vi "uTTA_GetLiveMeasureStatus.vi"(4 "CH1&2 Offset Voltage":dbl format="%.3pV", 6 "CH0 Offset Voltage":dbl format="%.3pV", 7 "uTTA_CalData":T1(array[cluster]), 8 "error in":errorcluster, 9 "CalibrationMode":bool, 10 "Timeout(ms)":i32=1000, 11 "VISA Refnum in":refnum<visa-resource-name>) -> (0 "error out":errorcluster, 1 "Measurement Completed":bool, 2 "Received":string, 3 "VISA Refnum out":refnum<visa-resource-name>, 5 "Measurement Data":T3)   [LabVIEW 2021]
uses:
  uTTA_Device_Driver/uTTA_Controls/CTL_uTTA_MeasurementStates.ctl
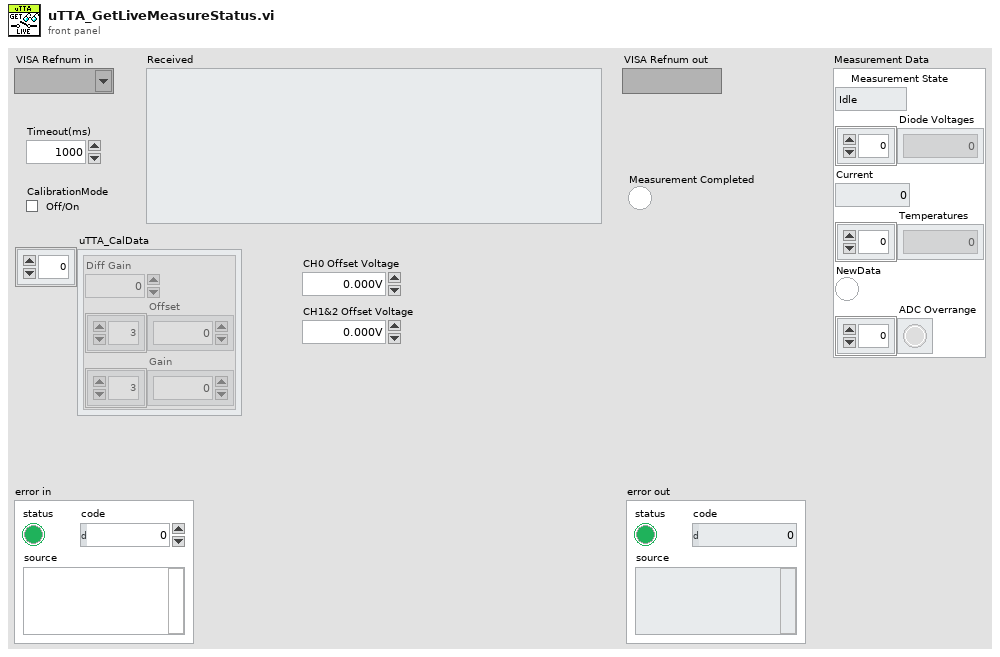
[diagram p1: front panel]
types:
  T1 = cluster{"Diff Gain":dbl, "Offset":dbl[], "Gain":dbl[]}[]
  T2 = typedef "CTL_uTTA_MeasurementStates.ctl" = enum16{"Idle", "Init", "GPPowerCheck", "InitMeasFile", "Preheating", "PrepHeating", "Heating", "PrepCooling", "Cooling", "Deinit", "CloseLog", "Cal_Init", "Cal_GDPowerOn", "Cal_GDPowerCheck", "Cal_Cal", "Cal_Deinit"}
  T3 = cluster{"Measurement State":T2, "Diode Voltages":dbl[], "Current":dbl, "Temperatures":dbl[], "NewData":bool, "ADC Overrange":bool[]}
  T4 = cluster{"Diff Gain":dbl, "Offset":dbl[], "Gain":dbl[]}
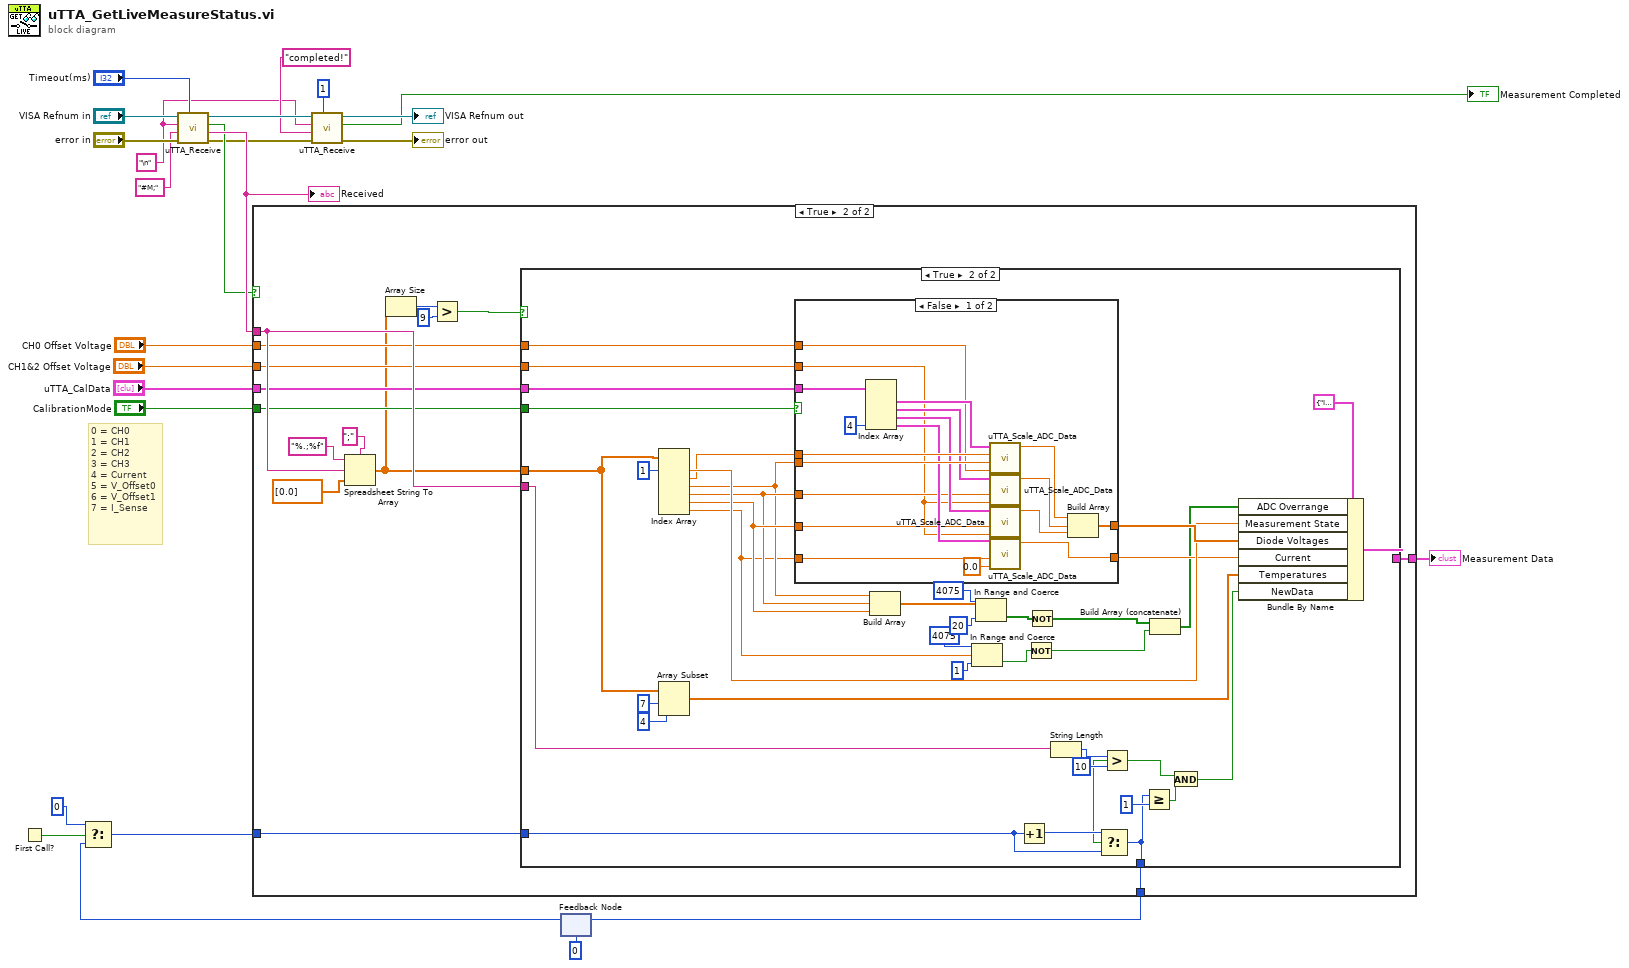
[diagram p0: block diagram]
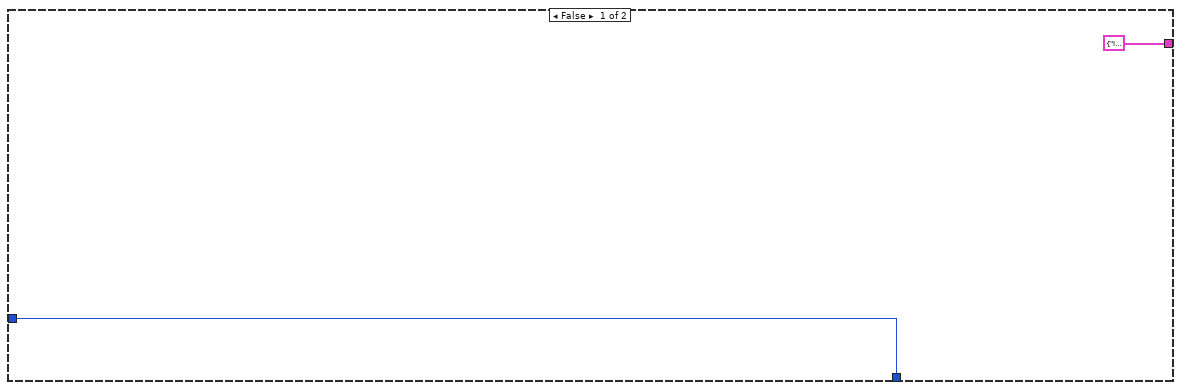
[diagram p2: hidden frame]
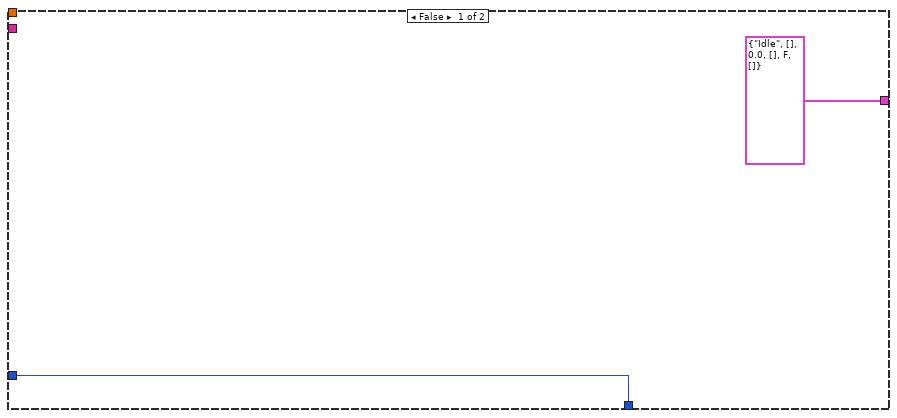
[diagram p3: hidden frame]
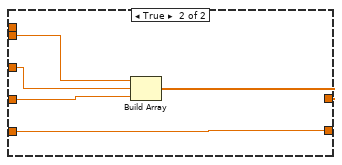
[diagram p4: hidden frame]
diagram:
  w1 = "\n" ("RX Termination(\\n)")
  # "0 = CH0\n1 = CH1\n2 = CH2\n3 = CH3\n4 = Current\n5 = V_Offset0\n6 = V_Offset1\n7 = I_Sense"
  n1 = First Call?() -> (First Call?: T/F=w19:bool)
  n2 = call "uTTA_Receive.vi"("Timeout(ms)"="Timeout(ms)", "error in (no error)"="error in", "Response Qualifier(\"\")"="#M;" ("Response Qualifier(\"\")"), "RX Termination(\\n)"=w1, "VISA Refnum in"="VISA Refnum in") -> ("error out"=w6:errorcluster, "Response"=w11:string, "Found response"=w9:bool, "VISA Refnum out"=w8:refnum<visa-resource-name>)  [unwired: 3 in]
  "Received" <- w11
  n3 = call "uTTA_Receive.vi"("Timeout(ms)"=1, "error in (no error)"=w6, "Response Qualifier(\"\")"="completed!" ("search string"), "RX Termination(\\n)"=w1, "VISA Refnum in"=w8) -> ("error out"=→"error out":errorcluster, "Found response"=→"Measurement Completed":bool, "VISA Refnum out"=→"VISA Refnum out":refnum<visa-resource-name>)  [unwired: 3 in, 1 out]
  n4 = feedback #1(0) -> (w18:i32)
  n5 = Select(t=0, s=w19, f=w18) -> (s? t:f=w17:i32)
  n6 = case shown="True" w9 {
    tunnel: w11 -> [_ w42]
    tunnel: [T3 {"Measurement State"=enum."Idle", "Diode Voltages"=[], "Current"=0.0, "Temperatures"=[], "NewData"=FALSE, "ADC Overrange"=[]} w40] -> w25
    tunnel: "CalibrationMode" -> [_ w41]
    tunnel: "uTTA_CalData" -> [_ w39]
    tunnel: "CH0 Offset Voltage" -> [_ w38]
    tunnel: "CH1&2 Offset Voltage" -> [_ w37]
    tunnel: w17 -> [w26 w36]
    tunnel: [w26 w35] -> w16
    frame False {
    }
    frame True {
      n7 = Spreadsheet String To Array(delimiter (Tab)=";", format string="%.;%f", spreadsheet string=w42, array type (2D Dbl)=dbl[] [0.0]) -> (array=w29:dbl[])
      n8 = Array Size(array=w29) -> (size(s)=w31:i32)
      n9 = Greater?(x=w31, y=9) -> (0:w28:bool)
      n10 = case shown="True" w28 {
        tunnel: [T3 {"Measurement State"=enum."Idle", "Diode Voltages"=[], "Current"=0.0, "Temperatures"=[], "NewData"=FALSE, "ADC Overrange"=[]} w79] -> w40
        tunnel: w42 -> [_ w72]
        tunnel: w41 -> [_ w70]
        tunnel: w39 -> [_ w65]
        tunnel: w38 -> [_ w64]
        tunnel: w37 -> [_ w63]
        tunnel: w36 -> [w43 w53]
        tunnel: [w43 w52] -> w35
        tunnel: w29 -> [_ w48]
        frame False {
        }
        frame True {
          n11 = Index Array(array=w48, index #1=1 ("index")) -> (element #1=w80:dbl, element #2=w71:dbl, element #3=w73:dbl, element #4=w74:dbl, element #5=w75:dbl, element #6=w59:dbl)  [unwired: 5 in]
          n12 = Array Subset(array=w48, index=7, length=4) -> (w45:dbl[])
          n13 = case shown="False" w70 {
            tunnel: [w102 w107] -> w81
            tunnel: [w87 w103] -> w76
            tunnel: w59 -> [w90 w103]
            tunnel: w75 -> [w91 w104]
            tunnel: w74 -> [w92 w105]
            tunnel: w73 -> [w100 w106]
            tunnel: w71 -> [w101 _]
            tunnel: w65 -> [w98 _]
            tunnel: w64 -> [w86 _]
            tunnel: w63 -> [w84 _]
            frame False {
              n14 = Index Array(array=w98, index #4=4 ("index")) -> (element #1=w97:T4, element #2=w96:T4, element #3=w95:T4, element #4=w94:T4)  [unwired: 3 in]
              n15 = call "uTTA_Scale_ADC_Data.vi"("Offset Voltage"=w86, "ADC Value"=w100, "PGA Setting"=w101, "Calibration"=w97) -> ("Scaled Output"=w99:dbl)  [unwired: 3 in]
              n16 = call "uTTA_Scale_ADC_Data.vi"("Offset Voltage"=w84, "ADC Value"=w92, "Calibration"=w96) -> ("Scaled Output"=w89:dbl)  [unwired: 4 in]
              n17 = call "uTTA_Scale_ADC_Data.vi"("Offset Voltage"=w84, "ADC Value"=w91, "Calibration"=w95) -> ("Scaled Output"=w88:dbl)  [unwired: 4 in]
              n18 = call "uTTA_Scale_ADC_Data.vi"("Offset Voltage"=0.0, "ADC Value"=w90, "Calibration"=w94) -> ("Scaled Output"=w87:dbl)  [unwired: 4 in]
              n19 = Build Array(w99, w89, w88) -> (w102:dbl[])
            }
            frame True {
              n20 = Build Array(w106, w105, w104) -> (w107:dbl[])
            }
          }
          n21 = Build Array(w73, w74, w75) -> (w68:dbl[])
          n22 = In Range and Coerce(upper limit=4075 ("index"), x=w59, lower limit=1 ("index")) -> (In Range?=w57:bool)  [unwired: 1 out]
          n23 = In Range and Coerce(upper limit=4075 ("index"), x=w68, lower limit=20 ("index")) -> (In Range?=w69:bool[])  [unwired: 1 out]
          n24 = Increment(x=w53) -> (x+1=w55:i32)
          n25 = Not(x=w57) -> (.not. x?=w58:bool)
          n26 = Not(x=w69) -> (.not. x?=w62:bool[])
          n27 = String Length(string=w72) -> (length=w78:i32)
          n28 = Greater?(x=w78, y=10) -> (0:w51:bool)
          n29 = Select(t=w55, s=w51, f=w53) -> (s? t:f=w52:i32)
          n30 = Greater Or Equal?(x=w52, y=1) -> (x >= y?=w50:bool)
          n31 = Build Array (concatenate)(w62, w58) -> (w56:bool[])
          n32 = And(x=w51, y=w50) -> (x .and. y?=w49:bool)
          n33 = Bundle By Name(cluster=T3 {"Measurement State"=enum."Idle", "Diode Voltages"=[], "Current"=0.0, "Temperatures"=[], "NewData"=TRUE, "ADC Overrange"=[]}, "ADC Overrange"=w56, "Measurement State"=w80, "Diode Voltages"=w81, "Current"=w76, "Temperatures"=w45, "NewData"=w49) -> (w79:T3)
        }
      }
    }
  }
  "Measurement Data" <- w25
  n34 = feedback-in #1(w16) -> ()
